vi "Move_Until_Home.vi"(8 "error in (no error)":errorcluster, 11 "VISA Refnum in":refnum<visa-resource-name>) -> (0 "error out":errorcluster, 3 "VISA Refnum out":refnum<visa-resource-name>)   [LabVIEW 2018]
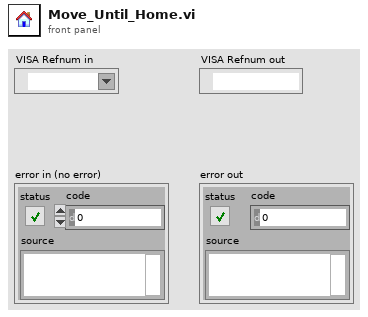
[diagram p1: front panel]
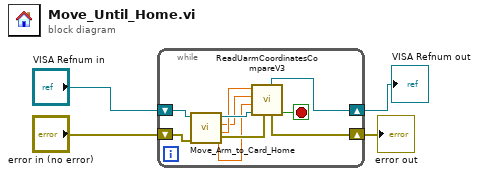
[diagram p0: block diagram]
diagram:
  n1 = while {
    shift-right: [w10] -> w3
    shift-left: "VISA Refnum in" -> [w14]
    shift-right: [w9] -> w4
    shift-left: "error in (no error)" -> [w13]
    stop <- w5 stop-if-true
    n2 = call "Move_Arm_to_Card_Home.vi"("error in"=w13, "Machine In"=w14) -> ("Z Coordinate"=w6:dbl, "Y Coordinate"=w8:dbl, "X Coordinate"=w7:dbl, "Machine Out"=w11:refnum<visa-resource-name>, "error out"=w12:errorcluster)  [unwired: 5 in]
    n3 = call "ReadUarmCoordinatesCompareV3.vi"("error in"=w12, "Machine In"=w11, "INPUT Z Coord"=w6, "INPUT X Coord"=w7, "INPUT Y Coord"=w8) -> ("x = y?"=w5:bool, "error out"=w9:errorcluster, "Machine Out"=w10:refnum<visa-resource-name>)  [unwired: 1 in, 3 out]
  }
  "error out" <- w4
  "VISA Refnum out" <- w3
